vi "Move.vi"(8 "error in (no error)":errorcluster, 9 "Absolute (T)":bool=TRUE, 10 "Point":refnum<class "Point.lvclass">, 11 "Square in":refnum<class "Square.lvclass">) -> (0 "error out":errorcluster, 3 "Square out":refnum<class "Square.lvclass">)   [LabVIEW 2021, in "Picture2D.lvlib" / "Square.lvclass"]
uses:
  Square.lvclass
  Square.lvclass/Square.ctl
  Rectangle/Rectangle.lvclass
  Point/Point.lvclass
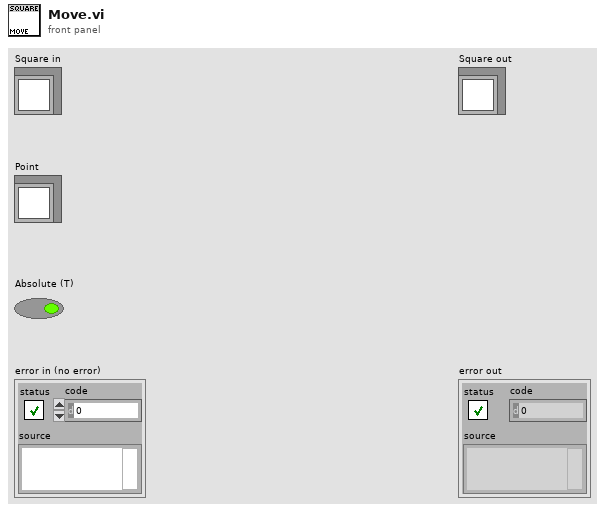
[diagram p1: front panel]
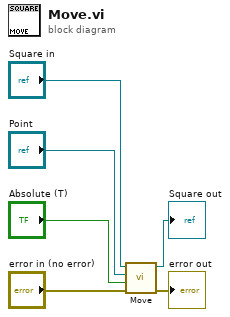
[diagram p0: block diagram]
diagram:
  n1 = call-parent "Move.vi"("error in (no error)"="error in (no error)", "Absolute (T)"="Absolute (T)", "Point"="Point", "Rectangle in"="Square in") -> ("error out"=→"error out":errorcluster, "Rectangle out"=→"Square out":refnum<class "Square.lvclass">)  [unwired: 6 in]
